vi "KickTactic_Init.vi"(0 "object in":refnum<class "KickTactic.lvclass">, 5 "error in (no error)":errorcluster) -> (14 "object out":refnum<class "KickTactic.lvclass">, 19 "error out":errorcluster)   [LabVIEW 2023, in "KickTactic.lvclass"]
uses:
  KickTactic.lvclass
  C:/Users/ebert/Documents/codes/SSL/repo/SSL_AI/NewSTP/NewTactics/Tactic_v2_class/Tactic_v2.lvclass
  NewSTP/NewSkills/HaltSkill_v2_class/HaltSkill_v2.lvclass
  C:/Users/ebert/Documents/codes/SSL/repo/SSL_AI/NewSTP/NewSkills/Skill_v2_class/Skill_v2.lvclass
  KickToSkill_v2_class/KickToSkill_v2.lvclass
  AlignToKick_class/AlignToKick.lvclass
  NewSTP/NewTactics/Tactic_v2_class/Tactic_v2.lvclass
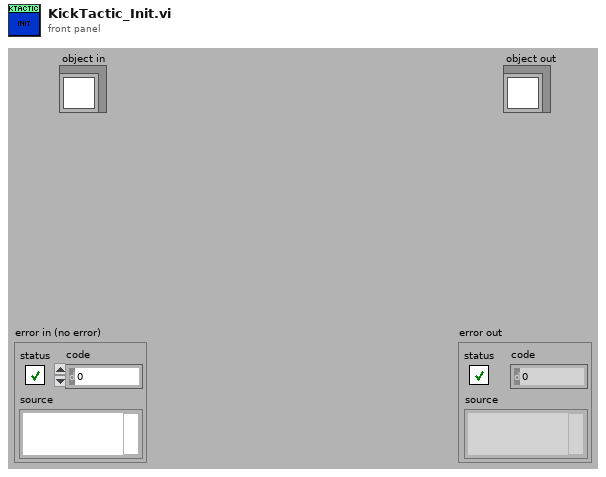
[diagram p1: front panel]
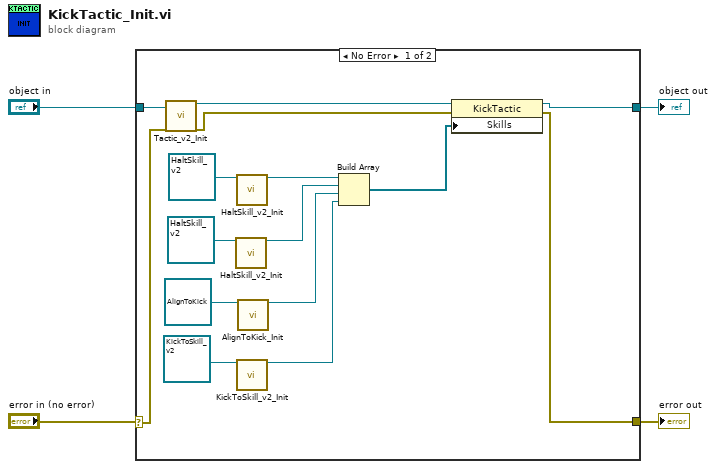
[diagram p0: block diagram]
diagram:
  n1 = case shown="No Error" "error in (no error)" {
    selector: "error in (no error)" -> [w9 w20]
    tunnel: [w10 w21] -> w4
    tunnel: "object in" -> [w19 w21]
    tunnel: [w8 w20] -> w1
    frame No Error {
      n2 = call "Tactic_v2_Init.vi"("object in"=w19, "error in (no error)"=w9) -> ("object out"=w18:refnum<class "KickTactic.lvclass">, "error out"=w5:errorcluster)  [unwired: 16 in]
      n3 = call "HaltSkill_v2_Init.vi"("object in"=refnum<class "HaltSkill_v2.lvclass"> refnum ("HaltSkill_v2")) -> ("object out"=w14:refnum<class "HaltSkill_v2.lvclass">)  [unwired: 17 in, 1 out]
      n4 = call "HaltSkill_v2_Init.vi"("object in"=refnum<class "HaltSkill_v2.lvclass"> refnum ("HaltSkill_v2")) -> ("object out"=w16:refnum<class "HaltSkill_v2.lvclass">)  [unwired: 17 in, 1 out]
      n5 = call "KickToSkill_v2_Init.vi"("object in"=refnum<class "KickToSkill_v2.lvclass"> refnum ("KickToSkill_v2")) -> ("object out"=w12:refnum<class "KickToSkill_v2.lvclass">)  [unwired: 17 in, 1 out]
      n6 = call "AlignToKick_Init.vi"("object in"=refnum<class "AlignToKick.lvclass"> refnum ("InterceptBallSkill")) -> ("object out"=w6:refnum<class "AlignToKick.lvclass">)  [unwired: 17 in, 1 out]
      n7 = Build Array(w16, w14, w6, w12) -> (w11:refnum<class "Skill_v2.lvclass">[])
      n8 = property class="KickTactic"(reference=w18, error in=w5, "Skills"=w11) -> (reference out=w10:refnum<class "KickTactic.lvclass">, error out=w8:errorcluster)
    }
    frame Error {
    }
  }
  "object out" <- w4
  "error out" <- w1
